vi "tutorial_03.vi"(2 "Temp Scale":bool) -> (0 "Thermometer":dbl(slide) scale=0.0..100.0)   [LabVIEW 2021]
uses:
  <vilib>/numeric/Random Number (Range) U64.vi
  <vilib>/numeric/sub_Random U32.vi
panel:
  # "Deg F"
  # "Deg C"
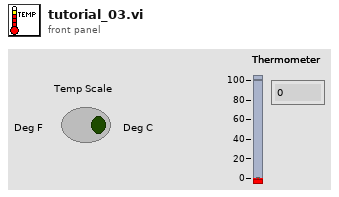
[diagram p1: front panel]
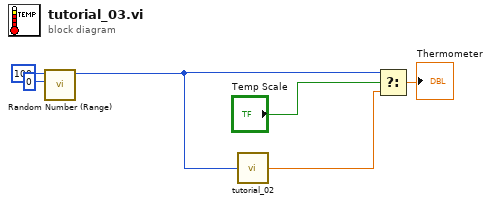
[diagram p0: block diagram]
diagram:
  n1 = call-poly <vilib>:"Random Number (Range).vi"("lower bound (0)"=u64 0, "upper bound (100)"=u64 100) -> ("number"=w3:u64)  [unwired: 9 in]
  n2 = call "tutorial_02.vi"("Deg C"=w3) -> ("Deg F"=w4:dbl)
  n3 = Select(t=w3, s="Temp Scale", f=w4) -> (s? t:f=→"Thermometer":dbl)
